vi "MOVTest.vi"() -> ()   [LabVIEW 2013]
uses:
  <vilib>/Instr/_visa.llb/VISA Configure Serial Port (Instr).vi
panel:
  out "POS? 2":string
  in  "Boolean":bool
  out "ERR?":string
  in  "VISA resource name":refnum<visa-resource-name>
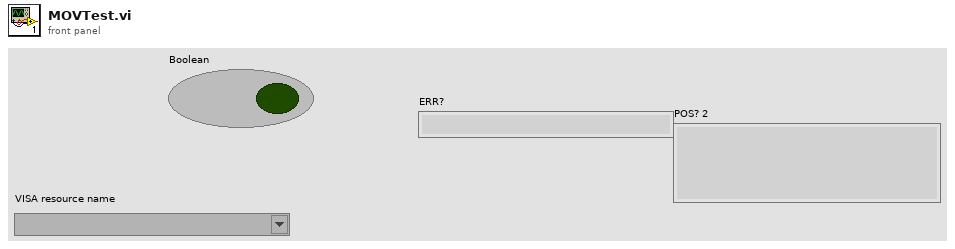
[diagram p1: front panel]
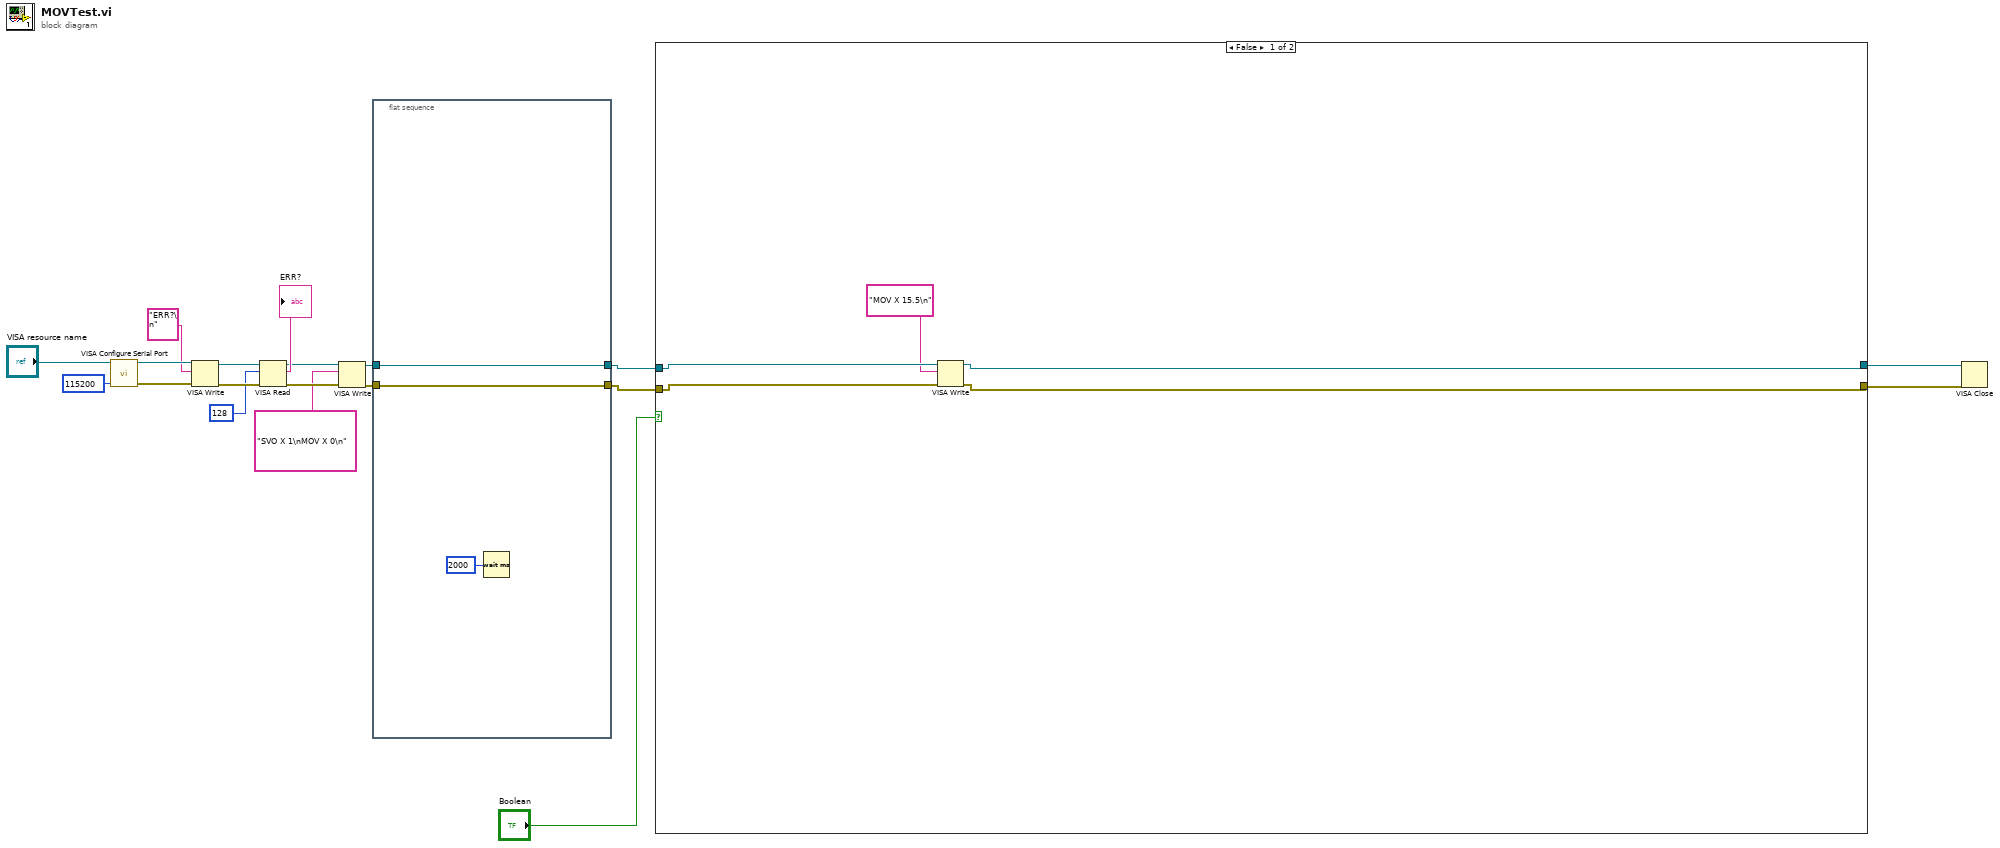
[diagram p0: block diagram]
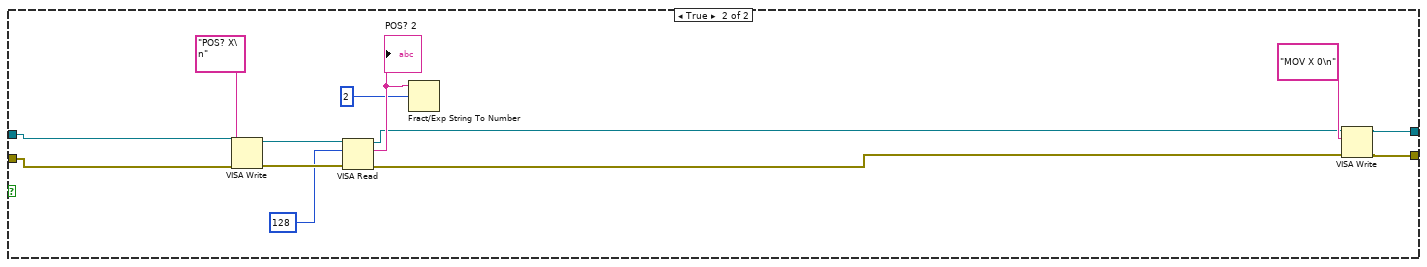
[diagram p2: hidden frame]
diagram:
  n1 = call-poly "VISA Configure Serial Port"("VISA resource name"="VISA resource name", "baud rate (9600)"=u32 115200) -> ("VISA resource name out"=w17:refnum<visa-resource-name>, "error out"=w16:errorcluster)  [unwired: 12 in]
  n2 = VISA Write(VISA resource name=w17, write buffer="ERR?\n", error in (no error)=w16) -> (VISA resource name out=w14:refnum<visa-resource-name>, error out=w13:errorcluster)  [unwired: 1 out]
  n3 = VISA Read(VISA resource name=w14, byte count=u32 128, error in (no error)=w13) -> (VISA resource name out=w10:refnum<visa-resource-name>, read buffer=→"ERR?":string, error out=w9:errorcluster)  [unwired: 1 out]
  n4 = VISA Write(VISA resource name=w10, write buffer="SVO X 1\nMOV X 0\n", error in (no error)=w9) -> (VISA resource name out=w7:refnum<visa-resource-name>, error out=w6:errorcluster)  [unwired: 1 out]
  n5 = flat-sequence {
    tunnel: [w21] -> w2
    tunnel: w7 -> [w21]
    tunnel: [w20] -> w1
    tunnel: w6 -> [w20]
    frame #0 {
      n6 = Wait (ms)(milliseconds to wait=u32 2000) -> ()  [unwired: 1 out]
    }
  }
  n7 = case shown="False" "Boolean" {
    tunnel: w2 -> [w27 w31]
    tunnel: w1 -> [w26 w30]
    tunnel: [w25 w39] -> w5
    tunnel: [w24 w38] -> w4
    frame False {
      n8 = VISA Write(VISA resource name=w27, write buffer="MOV X 15.5\n", error in (no error)=w26) -> (VISA resource name out=w25:refnum<visa-resource-name>, error out=w24:errorcluster)  [unwired: 1 out]
    }
    frame True {
      n9 = VISA Write(VISA resource name=w31, write buffer="POS? X\n", error in (no error)=w30) -> (VISA resource name out=w37:refnum<visa-resource-name>, error out=w36:errorcluster)  [unwired: 1 out]
      n10 = VISA Read(VISA resource name=w37, byte count=u32 128, error in (no error)=w36) -> (VISA resource name out=w29:refnum<visa-resource-name>, read buffer=w33:string, error out=w28:errorcluster)  [unwired: 1 out]
      "POS? 2" <- w33
      n11 = Fract/Exp String To Number(string=w33, offset=2) -> ()  [unwired: 2 in, 2 out]
      n12 = VISA Write(VISA resource name=w29, write buffer="MOV X 0\n", error in (no error)=w28) -> (VISA resource name out=w39:refnum<visa-resource-name>, error out=w38:errorcluster)  [unwired: 1 out]
    }
  }
  n13 = VISA Close(VISA resource name=w5, error in (no error)=w4) -> ()  [unwired: 1 out]
